vi "Create.vi"(5 "Test Suites in":refnum<class "Test Suites.lvclass">, 8 "error in (no error)":errorcluster) -> (0 "error out":errorcluster, 3 "Test Suites":refnum<class "Test Suites.lvclass">)   [LabVIEW 2013, in "JUnit XML.lvlib" / "Test Suites.lvclass"]
doc: "Creates a new instance of the <B>Test Suites</B> class."
uses:
  Test Suites.lvclass
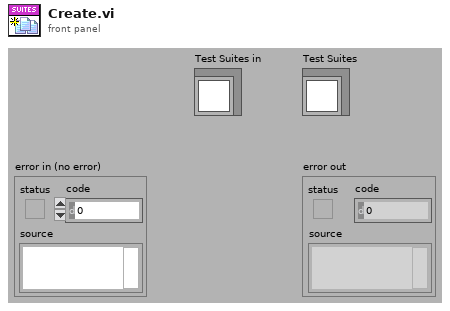
[diagram p1: front panel]
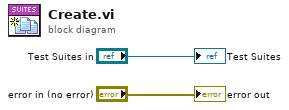
[diagram p0: block diagram]
diagram:
  "error out" <- "error in (no error)"
  "Test Suites" <- "Test Suites in"
